vi "Removed From Subpanel.vi"(8 "error in (no error)":errorcluster, 11 "IViewable in":refnum<class "IViewable.lvclass">) -> (0 "error out":errorcluster, 3 "IViewable out":refnum<class "IViewable.lvclass">)   [LabVIEW 2020, in "MVA Framework.lvlib" / "IViewable.lvlib" / "IViewable.lvclass"]
doc: "从子面板中删除"
uses:
  IViewable.lvclass
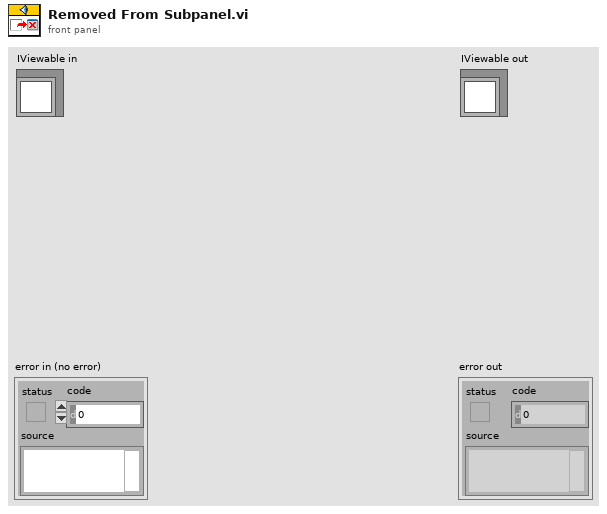
[diagram p1: front panel]
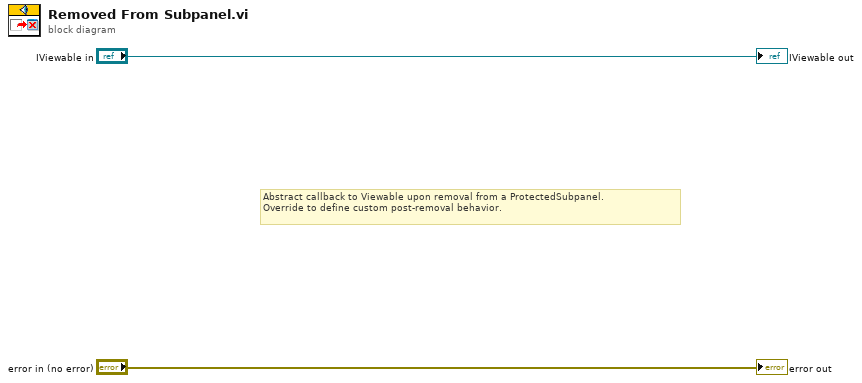
[diagram p0: block diagram]
diagram:
  # "Abstract callback to Viewable upon removal from a ProtectedSubpanel.\nOverride to define custom post-removal behavior."
  "error out" <- "error in (no error)"
  "IViewable out" <- "IViewable in"
